vi "Read Observer Reference.vi"(8 "error in (no error)":errorcluster, 11 "Device Connector in":refnum<class "Device Connector.lvclass">) -> (0 "error out":errorcluster, 2 "Observer Queue":T1, 3 "Device Connector out":refnum<class "Device Connector.lvclass">)   [LabVIEW 2024, in "Device Connector.lvclass"]
uses:
  Device Connector.lvclass
  Type Def/Observer Queue.ctl
  Ancestor Class/Actor Assistant/Observer/Observer.lvclass
  Device Connector.lvclass/Device Connector.ctl
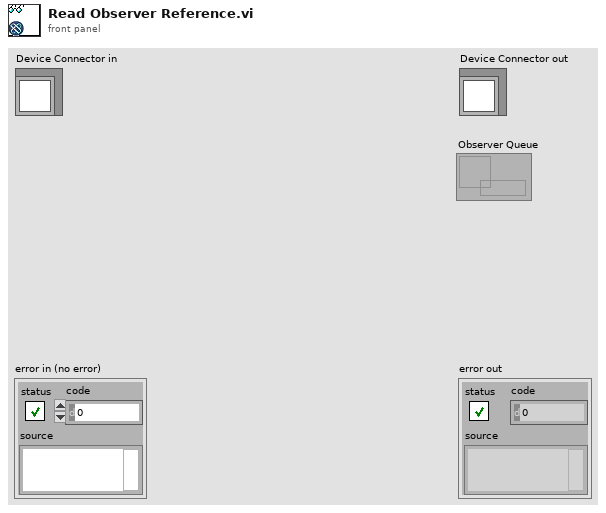
[diagram p1: front panel]
types:
  T1 = typedef "Observer Queue.ctl" = refnum<queue>
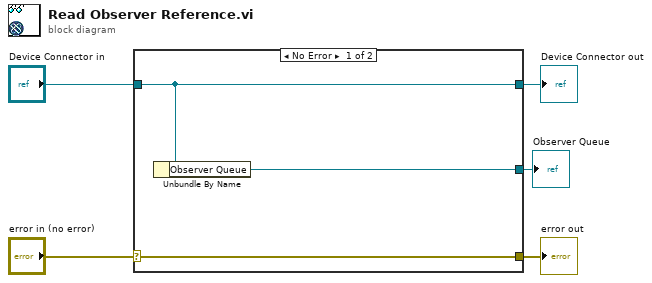
[diagram p0: block diagram]
diagram:
  n1 = case shown="No Error" "error in (no error)" {
    selector: "error in (no error)" -> [w8 w9]
    tunnel: [w8 w9] -> w4
    tunnel: [w7 w10] -> w2
    tunnel: "Device Connector in" -> [w7 w10]
    tunnel: [w6 _] -> w1
    frame No Error {
      n2 = Unbundle By Name(w7) -> ("Observer Queue"=w6:T1)
    }
    frame Error {
    }
  }
  "error out" <- w4
  "Device Connector out" <- w2
  "Observer Queue" <- w1
